vi "Write Element of Tree.vi"(8 "error in (no error)":errorcluster, 9 "Node":T1={"Record Type"="", "Payload"="", "Parent Index"=-1, "First Child Index"=-1, "Next Sibling Index"=-1}, 10 "index":i32, 11 "Fast Tree in":refnum<class "Fast Tree.lvclass">) -> (0 "error out":errorcluster, 3 "Fast Tree out":refnum<class "Fast Tree.lvclass">)   [LabVIEW 2019, in "Fast Tree.lvclass"]
uses:
  Fast Tree.lvclass
  Fast Tree.lvclass/Fast Tree.ctl
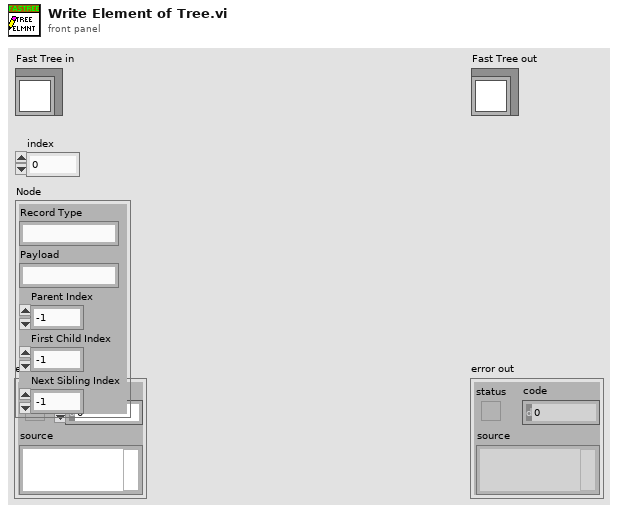
[diagram p1: front panel]
types:
  T1 = cluster{"Record Type":string, "Payload":string, "Parent Index":i32, "First Child Index":i32, "Next Sibling Index":i32}
  T2 = cluster{"Record Type":string, "Payload":string, "Parent Index":i32, "First Child Index":i32, "Next Sibling Index":i32}[]
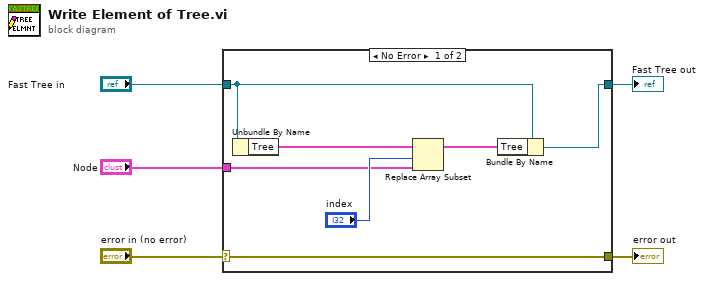
[diagram p0: block diagram]
diagram:
  n1 = case shown="No Error" "error in (no error)" {
    selector: "error in (no error)" -> [w12 w13]
    tunnel: [w12 w13] -> w4
    tunnel: [w11 w14] -> w2
    tunnel: "Fast Tree in" -> [w10 w14]
    tunnel: "Node" -> [w6 _]
    frame No Error {
      n2 = Unbundle By Name(w10) -> ("Tree"=w9:T2)
      n3 = Replace Array Subset(array=w9, new element=w6, index="index") -> (w8:T2)
      n4 = Bundle By Name(cluster=w10, "Tree"=w8) -> (w11:refnum<class "Fast Tree.lvclass">)
    }
    frame Error {
    }
  }
  "error out" <- w4
  "Fast Tree out" <- w2
